vi "set group poperty.vi"(0 "VISA in":refnum<visa-resource-name>, 5 "Group":string, 7 "Property":T1, 9 "Value to set":dbl min=0.0 max=1.0 step=1e-08 format="%.3pA", 11 "error in":errorcluster) -> (4 "VISA out":refnum<visa-resource-name>, 15 "error out":errorcluster)   [LabVIEW 2018]
uses:
  Group Properties.ctl
  CAEN globals.vi
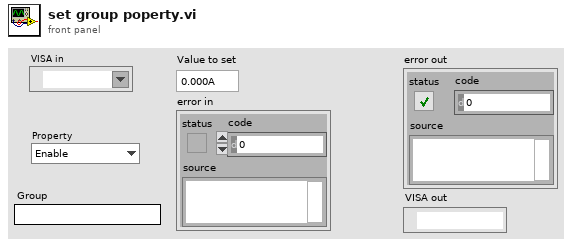
[diagram p1: front panel]
types:
  T1 = typedef "Group Properties.ctl" = enum16{"Enable", "Vset", "Imax", "Vswmax", "Trip Time"}
  T2 = typedef "channel.ctl" = cluster{" Card.Channel":dbl, "Crate":i32}
  T3 = cluster{"Group Name":string, "Channels in Group":T2[]}[]
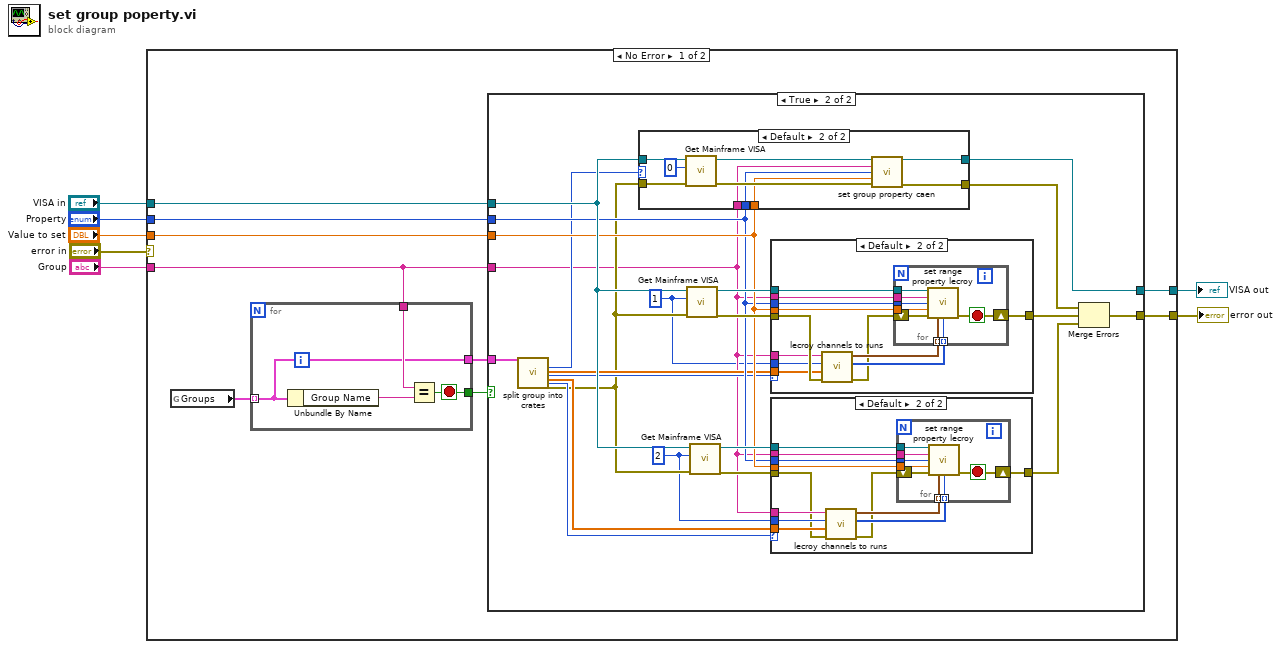
[diagram p0: block diagram]
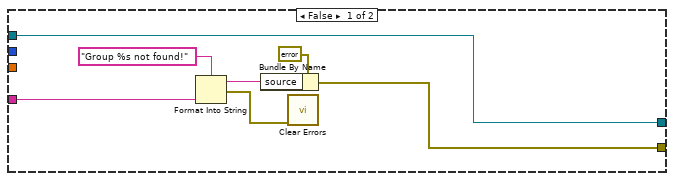
[diagram p2: hidden frame]
diagram:
  n1 = case shown="No Error" "error in" {
    selector: "error in" -> [_ w103]
    tunnel: [w14 w103] -> w7
    tunnel: "Property" -> [w13 _]
    tunnel: "VISA in" -> [w12 w102]
    tunnel: "Group" -> [w11 _]
    tunnel: "Value to set" -> [w10 _]
    tunnel: [w9 w102] -> w2
    frame No Error {
      n2 = global read "CAEN globals.vi" "Groups"() -> (w16:T3)
      n3 = for {
        tunnel: w16 -> [w98] mode=indexing
        tunnel: w11 -> [w100]
        tunnel: [w99] -> w15
        tunnel: [w98] -> w8
        stop <- w99 stop-if-true
        n4 = Unbundle By Name(w98) -> ("Group Name"=w101:string)
        n5 = Equal?(x=w100, y=w101) -> (x = y?=w99:bool)
      }
      n6 = case shown="True" w15 {
        tunnel: [w19 w35] -> w14
        tunnel: w13 -> [_ w37]
        tunnel: w12 -> [w17 w41]
        tunnel: w11 -> [w18 w25]
        tunnel: w10 -> [_ w38]
        tunnel: [w17 w33] -> w9
        tunnel: w8 -> [_ w45]
        frame False {
          n7 = Format Into String(format string="Group %s not found!" ("source"), w18) -> (resulting string=w23:string, error out=w20:errorcluster)  [unwired: 2 in]
          n8 = Bundle By Name(cluster=errorcluster {"status"=TRUE, "code"=0, "source"="Group %s not found!"} ("error out"), "source"=w23) -> (w19:errorcluster)
          n9 = call <vilib>:"Clear Errors.vi"("error in (no error)"=w20) -> ()  [unwired: 5 in, 2 out]
        }
        frame True {
          w24 = 1 ("Crate")
          w26 = 2 ("Crate")
          n10 = call "split group into crates.vi"("Group"=w45) -> ("Num Channels in Crate 0"=w32:i32, "Channels in Crate 1"=w30:dbl[], "Num Channels in Crate 1"=w31:i32, "Channels in Crate 2"=w28:dbl[], "Num Channels in Crate 2"=w29:i32, "error out"=w27:errorcluster)  [unwired: 19 in, 2 out]
          n11 = case shown="Default" w32 {
            tunnel: [w86 w95] -> w44
            tunnel: w41 -> [w87 w94]
            tunnel: w27 -> [w86 w93]
            tunnel: w25 -> [_ w92]
            tunnel: w38 -> [_ w91]
            tunnel: w37 -> [_ w90]
            tunnel: [w87 w89] -> w33
            frame 0 {
            }
            frame Default {
              n12 = call "Get Mainframe VISA.vi"("Error In"=w93, "Crate"=0, "VISA In"=w94) -> ("Error Out"=w96:errorcluster, "VISA out"=w97:refnum<visa-resource-name>)  [unwired: 6 in, 1 out]
              n13 = call "set group property caen.vi"("VISA in"=w97, "Group"=w92, "Property"=w90, "Value to set"=w91, "error in"=w96) -> ("VISA out"=w89:refnum<visa-resource-name>, "error out"=w95:errorcluster)  [unwired: 8 in, 1 out]
            }
          }
          n14 = call "Get Mainframe VISA.vi"("Error In"=w27, "Crate"=w24, "VISA In"=w41) -> ("Error Out"=w40:errorcluster, "VISA out"=w43:refnum<visa-resource-name>)  [unwired: 6 in, 1 out]
          n15 = call "Get Mainframe VISA.vi"("Error In"=w27, "Crate"=w26, "VISA In"=w41) -> ("Error Out"=w39:errorcluster, "VISA out"=w42:refnum<visa-resource-name>)  [unwired: 6 in, 1 out]
          n16 = case shown="Default" w31 {
            tunnel: [_ w77] -> w36
            tunnel: w43 -> [_ w76]
            tunnel: w40 -> [_ w69]
            tunnel: w25 -> [_ w75]
            tunnel: w38 -> [_ w74]
            tunnel: w37 -> [_ w73]
            tunnel: w30 -> [_ w67]
            tunnel: w25 -> [_ w68]
            tunnel: w24 -> [_ w66]
            frame 0 {
            }
            frame Default {
              n17 = call "lecroy channels to runs.vi"("error in"=w69, "Channels in Group"=w67, "Crate"=w66, "Group Name"=w68) -> ("error out"=w70:errorcluster, "Num Channels"=w71:i32[], "First Channel"=w72:T2[])  [unwired: 5 in]
              n18 = for {
                tunnel: w76 -> [w85]
                tunnel: w73 -> [w82]
                tunnel: w74 -> [w83]
                shift-right: [w80] -> w77
                shift-left: w70 -> [w84]
                tunnel: w75 -> [w81]
                tunnel: w72 -> [w79] mode=indexing
                tunnel: w71 -> [w78] mode=indexing
                stop <- w80 stop-if-true
                n19 = call "set range property lecroy.vi"("VISA in"=w85, "Group"=w81, "Property"=w82, "Value"=w83, "error in"=w84, "First Channel"=w79, "Num Channels"=w78) -> ("error out"=w80:errorcluster)  [unwired: 7 in, 1 out]
              }
            }
          }
          n20 = case shown="Default" w29 {
            tunnel: w42 -> [_ w57]
            tunnel: w39 -> [_ w47]
            tunnel: w25 -> [_ w56]
            tunnel: w38 -> [_ w55]
            tunnel: w37 -> [_ w54]
            tunnel: [_ w53] -> w34
            tunnel: w28 -> [_ w50]
            tunnel: w26 -> [_ w49]
            tunnel: w25 -> [_ w48]
            frame 0 {
            }
            frame Default {
              n21 = call "lecroy channels to runs.vi"("error in"=w47, "Channels in Group"=w50, "Crate"=w49, "Group Name"=w48) -> ("error out"=w46:errorcluster, "Num Channels"=w51:i32[], "First Channel"=w52:T2[])  [unwired: 5 in]
              n22 = for {
                tunnel: w57 -> [w65]
                tunnel: w54 -> [w62]
                tunnel: w55 -> [w63]
                shift-right: [w60] -> w53
                shift-left: w46 -> [w64]
                tunnel: w56 -> [w61]
                tunnel: w52 -> [w59] mode=indexing
                tunnel: w51 -> [w58] mode=indexing
                stop <- w60 stop-if-true
                n23 = call "set range property lecroy.vi"("VISA in"=w65, "Group"=w61, "Property"=w62, "Value"=w63, "error in"=w64, "First Channel"=w59, "Num Channels"=w58) -> ("error out"=w60:errorcluster)  [unwired: 7 in, 1 out]
              }
            }
          }
          n24 = Merge Errors(w44, w36, w34) -> (w35:errorcluster)
        }
      }
    }
    frame Error {
    }
  }
  "error out" <- w7
  "VISA out" <- w2
